vi "Generate Default CIF Project Name and Path.vi"(11 "MetaDataObj in":refnum<class "MetaDataObj.lvclass">) -> (1 "Project Root":path, 2 "Project Name":string, 3 "MetaDataObj out":refnum<class "MetaDataObj.lvclass">)   [LabVIEW 2021, in "CIF_Plugin_Generator.lvclass"]
uses:
  CIF_Plugin_Generator.lvclass
  <resource>/dialog/NewProjectWizard/MetaDataObj/MetaDataObj.lvclass
  <resource>/dialog/NewProjectWizard/MetaDataObj/MetaDataObj.lvclass/MetaDataObj.ctl
  <resource>/dialog/NewProjectWizard/MetaDataObj/Accessors/Write Project Root.vi
  <resource>/dialog/NewProjectWizard/MetaDataObj/Accessors/Write Project Name.vi
panel:
  # "Generate the libraries and classes needed for a new CIF plugin."
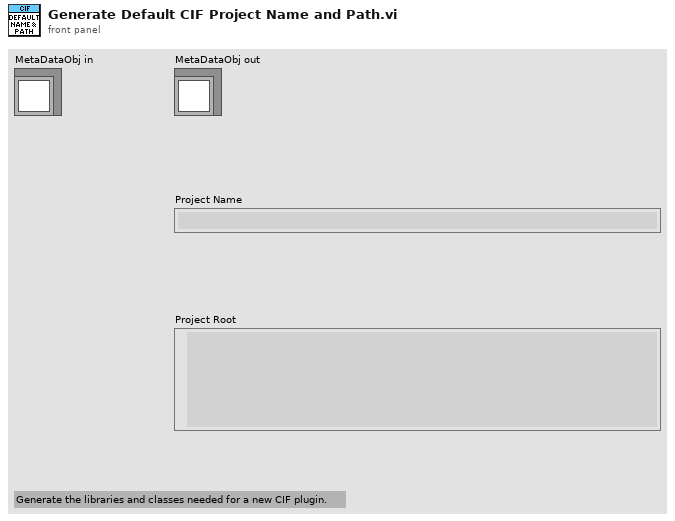
[diagram p1: front panel]
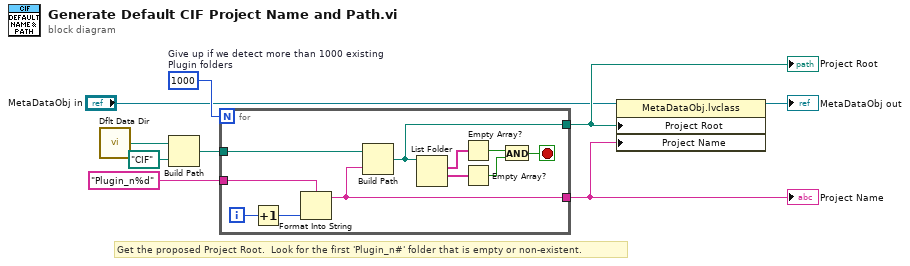
[diagram p0: block diagram]
diagram:
  w6 = 1000  # Give up if we detect more than 1000 existing Plugin folders
  # "Get the proposed Project Root.  Look for the first 'Plugin_n#' folder that is empty or non-existent."
  n1 = call <vilib>:"Dflt Data Dir.vi"() -> ("App:Default Data Directory"=w1:path)
  n2 = Build Path(base path=w1, name or relative path=path "CIF") -> (appended path=w3:path)
  n3 = for {
    N: w6 -> [_]
    tunnel: w3 -> [w20]
    tunnel: "Plugin_n%d" ("Untitled Project Name") -> [w19]
    tunnel: [w12] -> w8
    tunnel: [w11] -> w7
    i -> [w18]
    stop <- w10 stop-if-true
    n4 = Increment(x=w18) -> (x+1=w17:i32)
    n5 = Format Into String(format string=w19, w17) -> (resulting string=w12:string)  [unwired: 2 in, 1 out]
    n6 = Build Path(base path=w20, name or relative path=w12) -> (appended path=w11:path)
    n7 = List Folder(path=w11) -> (filenames=w16:string[], folder names=w15:string[])  [unwired: 3 in, 2 out]
    n8 = Empty Array?(array=w16) -> (empty?=w14:bool)
    n9 = Empty Array?(array=w15) -> (empty?=w13:bool)
    n10 = And(x=w14, y=w13) -> (x .and. y?=w10:bool)
  }
  "Project Name" <- w8
  "Project Root" <- w7
  n11 = property class="MetaDataObj.lvclass"(reference="MetaDataObj in", "Project Root"=w7, "Project Name"=w8) -> (reference out=→"MetaDataObj out":refnum<class "MetaDataObj.lvclass">)  [unwired: 1 in, 1 out]
